vi "Write Input Array.vi"(8 "error in (no error)":errorcluster, 10 "Input Array":u16[](array[numeric]), 11 "DtoA in":refnum<class "External Clock.lvclass">) -> (0 "error out":errorcluster, 3 "DtoA out":refnum<class "External Clock.lvclass">)   [LabVIEW 2014, in "External Clock.lvclass"]
uses:
  External Clock.lvclass
  External Clock.lvclass/External Clock.ctl
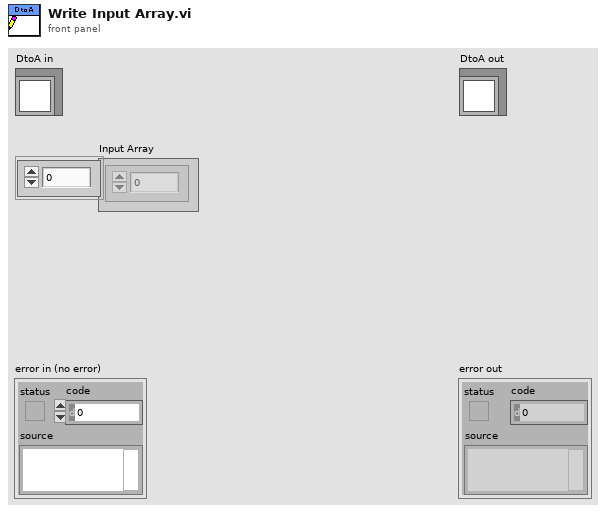
[diagram p1: front panel]
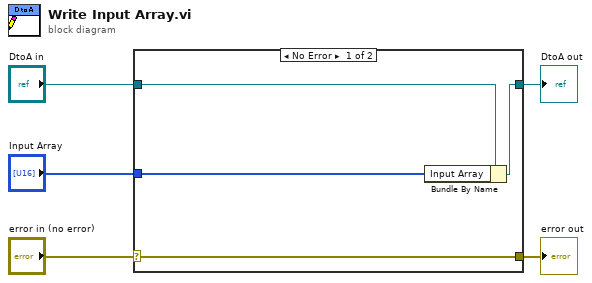
[diagram p0: block diagram]
diagram:
  n1 = case shown="No Error" "error in (no error)" {
    selector: "error in (no error)" -> [w9 w10]
    tunnel: [w9 w10] -> w4
    tunnel: [w7 w11] -> w2
    tunnel: "DtoA in" -> [w8 w11]
    tunnel: "Input Array" -> [w6 _]
    frame No Error {
      n2 = Bundle By Name(cluster=w8, "Input Array"=w6) -> (w7:refnum<class "External Clock.lvclass">)
    }
    frame Error {
    }
  }
  "error out" <- w4
  "DtoA out" <- w2
